vi "Str2HexStr.vi"(1 "数组大小":i32, 2 "数组":i8[](array[numeric]) format="%02x") -> (0 "OutStr":string)   [LabVIEW 2015]
doc: "将字符串分隔为无符号8位整形的数据，然后格式化为十六进制字符串，例 “YS_COM” --> \"59 53 5F 43 4F 4D \""
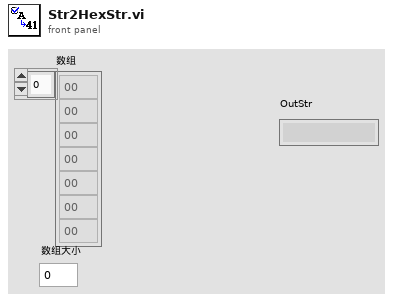
[diagram p1: front panel]
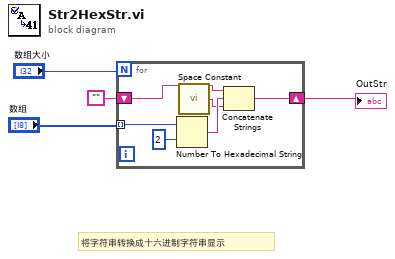
[diagram p0: block diagram]
diagram:
  # "将字符串转换成十六进制字符串显示"
  n1 = for {
    N: "数组大小" -> [_]
    tunnel: "数组" -> [w10] mode=indexing
    shift-right: [w9] -> w3
    shift-left: "" -> [w8]
    n2 = Number To Hexadecimal String(1:2, 2:w10) -> (0:w6:string)
    n3 = call <vilib>:"Space Constant.vi"() -> ("String"=w5:string)
    n4 = Concatenate Strings(w8, w6, w5) -> (w9:string)
  }
  "OutStr" <- w3
